vi "Calculate track length in samples.vi"(6 "Sample Rate (Hz)":dbl, 9 "Time Signature":enum16{"4/4", "3/4"}(ring), 10 "BPM":i32, 11 "Measures":i32) -> (0 "total number of beats":i32, 1 "bps":dbl, 2 "Track Length in Samples":i32, 3 "Track Division in Samples":i32)   [LabVIEW 2014]
uses:
  Controls/sample block size.vi
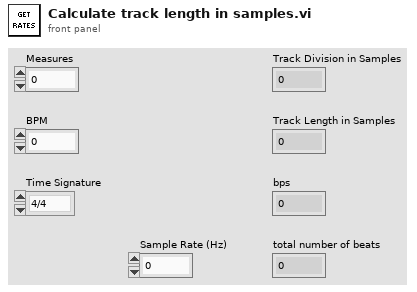
[diagram p1: front panel]
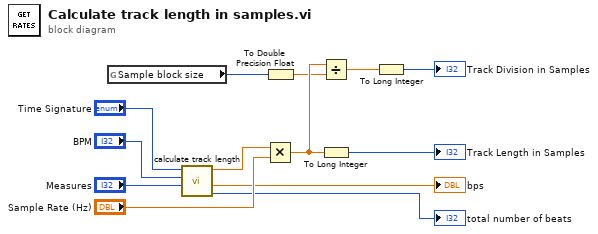
[diagram p0: block diagram]
diagram:
  n1 = global read "sample block size.vi" "Sample block size"() -> (w4:i32)
  n2 = call "calculate track length.vi"("Measures"="Measures", "BPM"="BPM", "Enum"="Time Signature") -> ("total number of beats"=→"total number of beats":i32, "bps"=→"bps":dbl, "Track Length (s)"=w5:dbl)  [unwired: 6 in]
  n3 = Multiply(x=w5, y="Sample Rate (Hz)") -> (x*y=w12:dbl)
  n4 = To Double Precision Float(number=w4) -> (double precision float=w3:dbl)
  n5 = Divide(x=w12, y=w3) -> (x/y=w7:dbl)
  n6 = To Long Integer(number=w12) -> (32bit integer=→"Track Length in Samples":i32)
  n7 = To Long Integer(number=w7) -> (32bit integer=→"Track Division in Samples":i32)
